vi "二值化阈值自动调节（二值版）.vi"(1 "当前阈值":dbl, 2 "允许损失":dbl, 3 "白点百分比（0-100）默认50":dbl, 4 "输入image数组（灰度）":dbl[][](array[numeric])) -> (0 "二值化阈值":dbl)   [LabVIEW 2017]
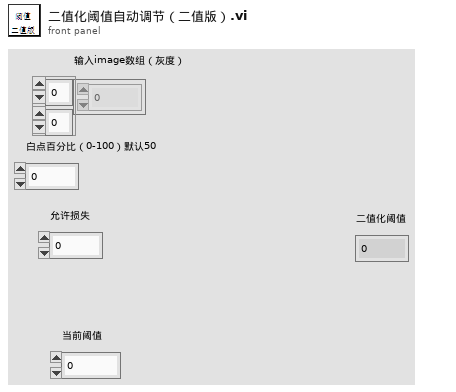
[diagram p1: front panel]
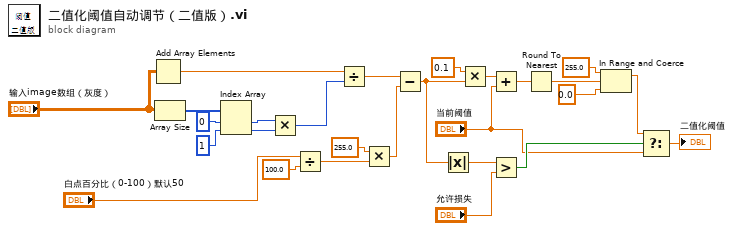
[diagram p0: block diagram]
diagram:
  n1 = Add Array Elements(numeric array="输入image数组（灰度）") -> (sum=w22:dbl)
  n2 = Array Size(array="输入image数组（灰度）") -> (size(s)=w27:i32[])
  n3 = Index Array(array=w27, index #1=0, index #2=1) -> (element #1=w24:i32, element #2=w23:i32)
  n4 = Multiply(x=w24, y=w23) -> (x*y=w20:i32)
  n5 = Divide(x="白点百分比（0-100）默认50", y=100.0) -> (x/y=w14:dbl)
  n6 = Divide(x=w22, y=w20) -> (x/y=w2:dbl)
  n7 = Multiply(x=255.0, y=w14) -> (x*y=w1:dbl)
  n8 = Subtract(x=w2, y=w1) -> (x-y=w4:dbl)
  n9 = Absolute Value(x=w4) -> (abs(x)=w3:dbl)
  n10 = Multiply(x=0.1, y=w4) -> (x*y=w8:dbl)
  n11 = Add(x=w8, y="当前阈值") -> (x+y=w6:dbl)
  n12 = Greater?(x=w3, y="允许损失") -> (0:w11:bool)
  n13 = Round To Nearest(number=w6) -> (nearest integer value=w17:dbl)
  n14 = In Range and Coerce(upper limit=255.0, x=w17, lower limit=0.0) -> (coerced(x)=w5:dbl)  [unwired: 1 out]
  n15 = Select(t=w5, s=w11, f="当前阈值") -> (s? t:f=→"二值化阈值":dbl)
